vi "speed regulation.vi"(10 "limit":dbl, 11 "up and down":dbl) -> (1 "output":dbl)   [LabVIEW 2016]
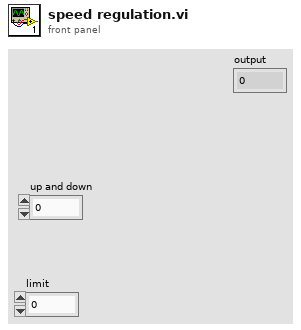
[diagram p1: front panel]
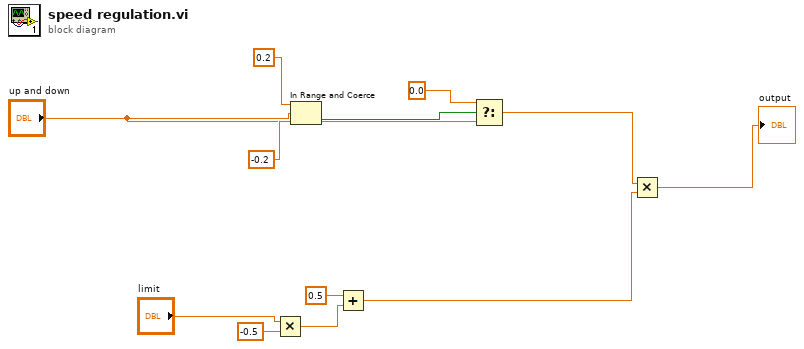
[diagram p0: block diagram]
diagram:
  n1 = Multiply(x="limit", y=-0.5) -> (x*y=w5:dbl)
  n2 = In Range and Coerce(upper limit=0.2, x="up and down", lower limit=-0.2) -> (In Range?=w10:bool)  [unwired: 1 out]
  n3 = Add(x=0.5, y=w5) -> (x+y=w3:dbl)
  n4 = Select(t=0.0, s=w10, f="up and down") -> (s? t:f=w2:dbl)
  n5 = Multiply(x=w2, y=w3) -> (x*y=→"output":dbl)
